vi "LC-MISDK_Meas_Lv_LOEM.vi"(0 ".NET reference":refnum<k24>, 5 "comPort":i32, 11 "error in":errorcluster) -> (4 ".NET reference out":refnum<k24>, 6 "Lv":dbl, 8 "Lv Display":dbl, 13 "ReadLatestData Error":dbl format="%#_6f", 15 "error out":errorcluster)   [LabVIEW 2019]
uses:
  C:/Program Files (x86)/National Instruments/LabVIEW 2019/LC-MISDK.dll
  Program Files (x86)/National Instruments/LabVIEW 2019/LC-MISDK.dll
panel:
  # "Reprogramado Por Fredy Osorio 05/2025\ning.fredyosorio@gmail.com\nhttps://github.com/fr3dyos/PUC-LOEM-Controle-Minolta"
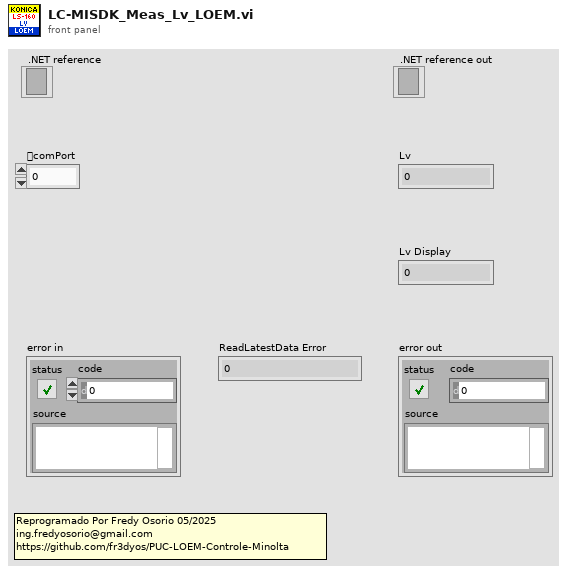
[diagram p1: front panel]
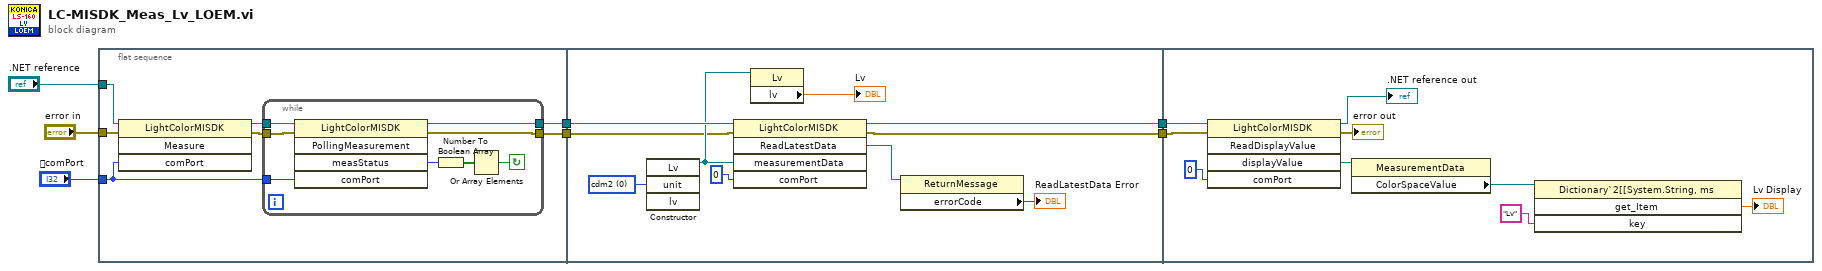
[diagram p0: block diagram]
diagram:
  n1 = flat-sequence {
    tunnel: ".NET reference" -> [w13]
    tunnel: "comPort" -> [w11]
    tunnel: [w14] -> w7
    tunnel: "error in" -> [w10]
    tunnel: [w8] -> w2
    tunnel: w7 -> [w31]
    tunnel: [w29] -> w3
    tunnel: w2 -> [w24]
    tunnel: [w23] -> w1
    tunnel: w3 -> [w41]
    tunnel: w1 -> [w34]
    frame #0 {
      n2 = invoke on="インボークノード" class="LightColorMISDK" method="Measure"(reference=w13, error in=w10, "comPort"=w11) -> (reference out=w12:refnum<k24>, error out=w9:errorcluster)  [unwired: 1 in, 2 out]
      n3 = while {
        tunnel: [w21] -> w14
        tunnel: w12 -> [w20]
        tunnel: w11 -> [w19]
        tunnel: w9 -> [w16]
        tunnel: [w15] -> w8
        stop <- w17 continue-if-true
        n4 = invoke on="インボークノード" class="LightColorMISDK" method="PollingMeasurement"(reference=w20, error in=w16, "comPort"=w19) -> (reference out=w21:refnum<k24>, error out=w15:errorcluster, "measStatus"=w22:i32)  [unwired: 2 in, 2 out]
        n5 = Number To Boolean Array(number=w22) -> (Boolean array=w18:bool[])
        n6 = Or Array Elements(Boolean array=w18) -> (logical OR=w17:bool)
      }
    }
    frame #1 {
      w27 = 0 items=["cdm2", "other"] ("unit")
      n7 = constructor class="Lv"("unit"=w27) -> (reference out=w26:refnum<k24>)  [unwired: 4 in, 4 out]
      n8 = invoke class="LightColorMISDK" method="ReadLatestData"(reference=w31, error in=w24, "measurementData"=w26, "comPort"=0) -> (reference out=w29:refnum<k24>, error out=w23:errorcluster, "ReadLatestData"=w28:refnum<k24>)  [unwired: 1 in, 2 out]
      n9 = property class="Lv"(reference=w26) -> ("lv"=→"Lv":dbl)  [unwired: 1 in, 2 out]
      n10 = property on="プロパティノード" class="ReturnMessage"(reference=w28) -> ("errorCode"=→"ReadLatestData Error":i32)  [unwired: 1 in, 2 out]
    }
    frame #2 {
      n11 = invoke class="LightColorMISDK" method="ReadDisplayValue"(reference=w41, error in=w34, "comPort"=0) -> (reference out=→".NET reference out":refnum<k24>, error out=→"error out":errorcluster, "displayValue"=w39:refnum<k24>)  [unwired: 2 in, 2 out]
      n12 = property class="MeasurementData"(reference=w39) -> ("ColorSpaceValue"=w36:refnum<k24>)  [unwired: 1 in, 2 out]
      n13 = invoke class="Dictionary`2[[System.String, ms" method="get_Item"(reference=w36, "key"="Lv") -> ("get_Item"=→"Lv Display":dbl)  [unwired: 2 in, 3 out]
    }
  }
